vi "Strip File Extension.vi"(11 "LVLIBP Name In":string) -> (3 "Library Name with Extension Stripped":string)   [LabVIEW 2019, in "NIPKG Naming.lvlib"]
uses:
  NIPKG Naming.lvlib
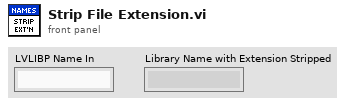
[diagram p1: front panel]
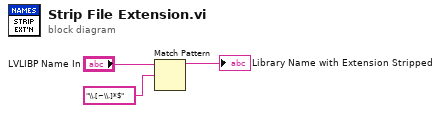
[diagram p0: block diagram]
diagram:
  n1 = Match Pattern(string="LVLIBP Name In", regular expression="\\.[~\\.]*$") -> (before substring=→"Library Name with Extension Stripped":string)  [unwired: 4 out]
